vi "Filter Wheel Template.vi"(0 "Notifier Name In":string, 2 "Wait for Finish":bool=TRUE, 11 "Error In":errorcluster) -> (4 "Notifier Name Out":string, 15 "Error Out":errorcluster)   [LabVIEW 2020]
uses:
  FW Type Defs/FW Notifier Type.ctl
  FW Type Defs/FW Actions.ctl
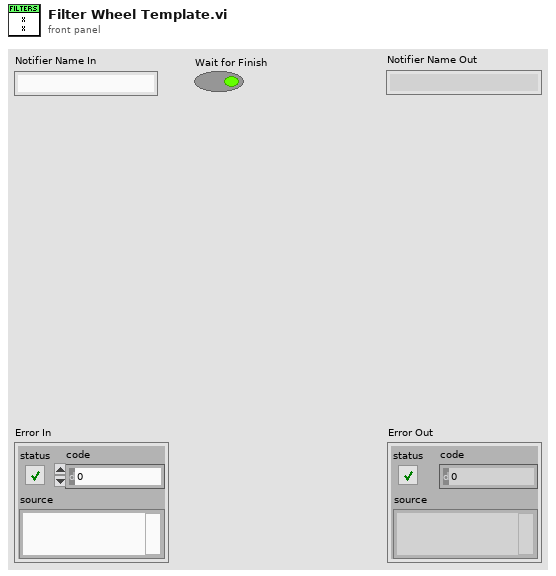
[diagram p1: front panel]
types:
  T1 = typedef "FW Notifier Type.ctl" = cluster{"Actions":T2, "Set Position":u8, "Actual Position":u8, "Speed":dbl, "Num Positions":u8, "Received":bool}
  T2 = typedef "FW Actions.ctl" = enum16{"Set Position", "Get Position", "Get Num Positions", "Set Speed", "Confirm Pos", "Quit"}
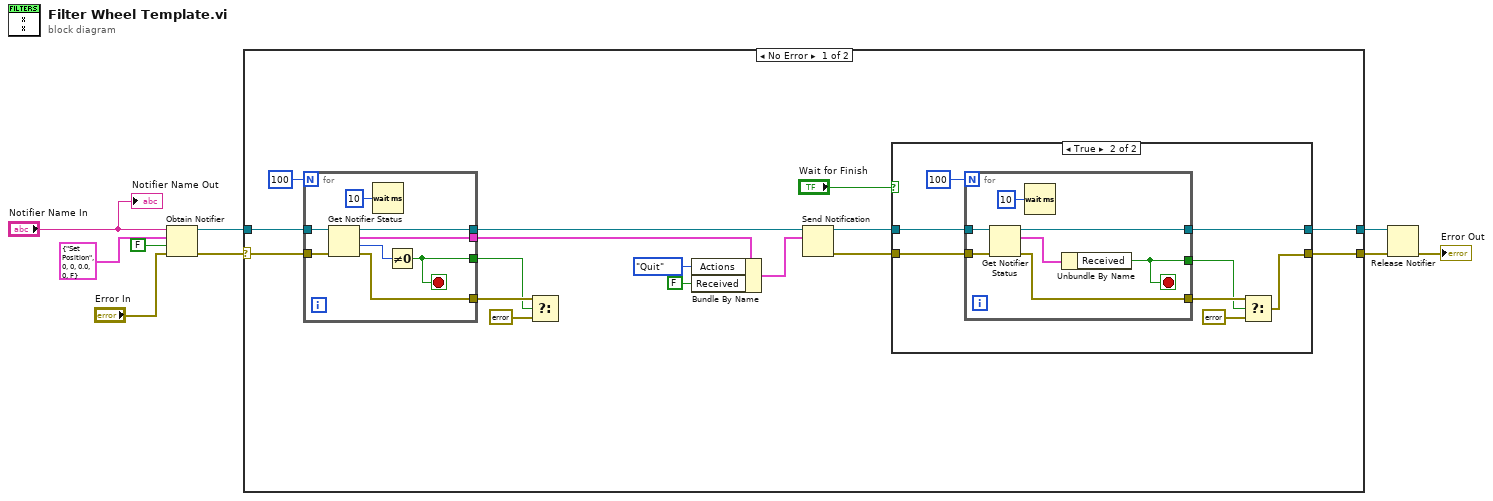
[diagram p0: block diagram]
diagram:
  n1 = Obtain Notifier(name (unnamed)="Notifier Name In", notification data type=T1 {"Actions"=enum."Set Position", "Set Position"=0, "Actual Position"=0, "Speed"=0.0, "Num Positions"=0, "Received"=FALSE} ("FW102C Note Type"), create if not found? (T)=FALSE, error in (no error)="Error In") -> (notifier out=w6:refnum<notifier>, error out=w7:errorcluster)  [unwired: 1 out]
  n2 = case shown="No Error" w7 {
    selector: w7 -> [w23 w52]
    tunnel: w6 -> [w25 w51]
    tunnel: [w17 w52] -> w3
    tunnel: [w18 w51] -> w4
    frame No Error {
      n3 = for {
        N: 100 -> [_]
        tunnel: w25 -> [w50]
        tunnel: [w48] -> w14
        tunnel: [w46] -> w22
        tunnel: w23 -> [w45]
        tunnel: [w44] -> w15
        tunnel: [w43] -> w10
        stop <- w48 stop-if-true
        n4 = Get Notifier Status(notifier=w50, error in (no error)=w45) -> (notifier out=w46:refnum<notifier>, current notification=w43:T1, # waiting=w49:i32, error out=w44:errorcluster)  [unwired: 1 out]
        n5 = Wait (ms)(milliseconds to wait=u32 10) -> ()  [unwired: 1 out]
        n6 = Not Equal To 0?(x=w49) -> (x != 0?=w48:bool)
      }
      n7 = Select(t=w15, s=w14, f=errorcluster {"status"=TRUE, "code"=0, "source"="Filter wheel busy. Timeout error."}) -> ()  [unwired: 1 out]
      n8 = Bundle By Name(cluster=w10, "Actions"=FW_Actions."Quit", "Received"=FALSE) -> (w21:T1)
      n9 = Send Notification(notification=w21, notifier=w22) -> (notifier out=w19:refnum<notifier>, error out=w20:errorcluster)  [unwired: 1 in]
      n10 = case shown="True" "Wait for Finish" {
        tunnel: w20 -> [w26 w35]
        tunnel: w19 -> [w27 w34]
        tunnel: [w27 w33] -> w18
        tunnel: [w26 w32] -> w17
        frame False {
        }
        frame True {
          n11 = for {
            N: 100 -> [_]
            tunnel: w34 -> [w42]
            tunnel: [w40] -> w33
            tunnel: w35 -> [w39]
            tunnel: [w38] -> w30
            tunnel: [w36] -> w29
            stop <- w36 stop-if-true
            n12 = Get Notifier Status(notifier=w42, error in (no error)=w39) -> (notifier out=w40:refnum<notifier>, current notification=w37:T1, error out=w38:errorcluster)  [unwired: 2 out]
            n13 = Wait (ms)(milliseconds to wait=u32 10) -> ()  [unwired: 1 out]
            n14 = Unbundle By Name(w37) -> ("Received"=w36:bool)
          }
          n15 = Select(t=w30, s=w29, f=errorcluster {"status"=TRUE, "code"=0, "source"="Filter Wheel Error: Action didn't complete."}) -> (s? t:f=w32:errorcluster)
        }
      }
    }
    frame Error {
    }
  }
  n16 = Release Notifier(notifier=w4, error in (no error)=w3) -> (error out=→"Error Out":errorcluster)  [unwired: 1 in, 2 out]
  "Notifier Name Out" <- "Notifier Name In"
